vi "Build Channel List Dual Channel.vi"(9 "Channel":string, 10 "Data line":u16, 11 "Protocol capture resource name":string) -> (3 "String":string)   [LabVIEW 2021, in "audio_adc_acDualChannelMeasurement.lvlib"]
uses:
  audio_adc_acDualChannelMeasurement.lvlib
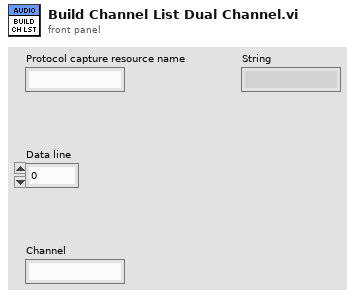
[diagram p1: front panel]
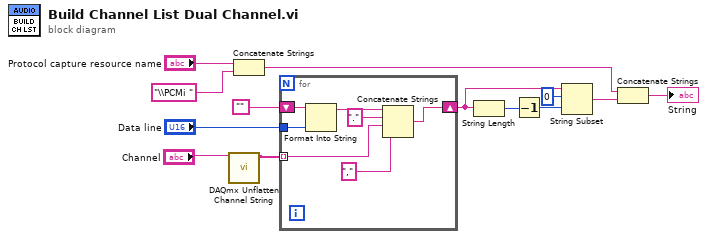
[diagram p0: block diagram]
diagram:
  n1 = call <vilib>:"DAQmx Unflatten Channel String.vi"("names in"="Channel") -> ("names out"=w9:string[])  [unwired: 13 in, 1 out]
  n2 = Concatenate Strings("Protocol capture resource name", "\\PCMi " ("string")) -> (w1:string)
  n3 = for {
    tunnel: "Data line" -> [w20]
    tunnel: w9 -> [w16] mode=indexing
    shift-right: [w14] -> w5
    shift-left: "" -> [w19]
    n4 = Format Into String(initial string=w19, w20) -> (resulting string=w18:string)  [unwired: 2 in, 1 out]
    n5 = Concatenate Strings(w18, "." ("string"), w16, "," ("string")) -> (w14:string)
  }
  n6 = String Length(string=w5) -> (length=w7:i32)
  n7 = Decrement(x=w7) -> (x-1=w6:i32)
  n8 = String Subset(string=w5, offset (0)=0, length (rest)=w6) -> (substring=w3:string)
  n9 = Concatenate Strings(w1, w3) -> (→"String":string)
